vi "ENPH 354 Assignment 1 - Q2.vi"() -> ()   [LabVIEW 2021]
panel:
  out "Array":dbl[][](array[numeric])
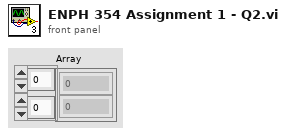
[diagram p1: front panel]
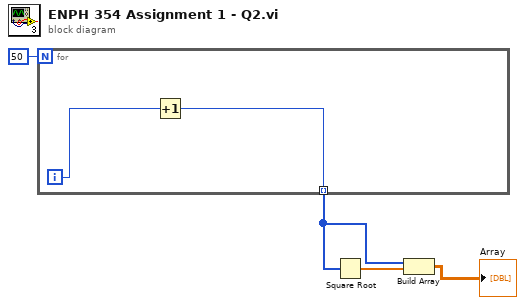
[diagram p0: block diagram]
diagram:
  n1 = for {
    N: 50 -> [_]
    tunnel: [w5] -> w2 mode=indexing
    i -> [w6]
    n2 = Increment(x=w6) -> (x+1=w5:i32)
  }
  n3 = Square Root(x=w2) -> (sqrt(x)=w3:dbl[])
  n4 = Build Array(w2, w3) -> (→"Array":dbl[][])
